vi "Disabled.vi"(7 "Robot Mode":T2, 10 "Match Info":T1={"Autonomous Elapsed Seconds"=0.0, "TeleOp Elapsed Seconds"=0.0, "Disabled Elapsed Seconds"=0.0, "Visited Autonomous"=FALSE, "Visited TeleOp"=FALSE, "Visited Disabled"=FALSE, "Autonomous Settings"={"Autonomous Style"=enum."Independent", "VI Refnum"=refnum}}, 11 "Call Context":T3) -> ()   [LabVIEW 2015]
doc: "This VI is called each time a disabled packet is received from the DS. It is often used to prepare for the next robot mode, to calibrate sensors, etc."
uses:
  <vilib>/Rock Robotics/WPI/DriverStation/WPI_DriverStationDerivedRobotMode.ctl
  <vilib>/Rock Robotics/WPI/DriverStation/WPI_DriverStationRobotMode2.ctl
  <vilib>/Rock Robotics/WPI/DriverStation/WPI_DriverStationMatch Info.ctl
  Drivetrain Code/Drivetrain Control.ctl
  Drivetrain Code/Drivetrain Mode.ctl
  Rollers/Roller Modes.ctl
  Common Code/Auto Roller Commands.ctl
  Common Code/Roller Mode Enum.ctl
  Elevator/Elevator Command.ctl
  Common Code/Change Detect Boolean.vi
  <vilib>/Rock Robotics/WPI/Utilities/WPI_GetSetVariantRefNum.vi
  Robot Global Data.vi
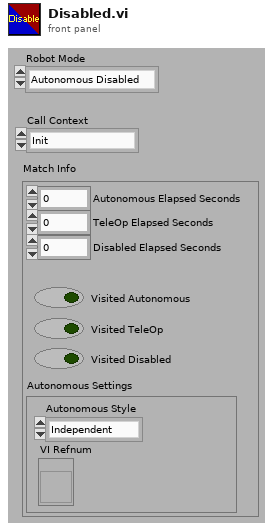
[diagram p1: front panel]
types:
  T1 = typedef "WPI_DriverStationMatch Info.ctl" = cluster{"Autonomous Elapsed Seconds":dbl, "TeleOp Elapsed Seconds":dbl, "Disabled Elapsed Seconds":dbl, "Visited Autonomous":bool, "Visited TeleOp":bool, "Visited Disabled":bool, "Autonomous Settings":cluster{"Autonomous Style":enum16{"Iterative", "Independent"}, "VI Refnum":refnum<vi>}}
  T2 = typedef "WPI_DriverStationRobotMode2.ctl" = enum16{"Autonomous Disabled", "Autonomous Enabled", "Teleop Disabled", "Teleop Enabled", "Disconnected", "Finish", "Test Disabled", "Test Enabled", "Emergency Stopped"}
  T3 = typedef "WPI_DriverStationDerivedRobotMode.ctl" = enum16{"Init", "Execute", "Stop"}
  T4 = enum16{"0", "1", "2", "3", "4", "5", "6", "7", "8", "9", "A", "B", "C", "D", "E", "F", "G", "H", "I", "J", "K", "L", "M", "N", "O", "P", "Q", "R", "S", "T", "U", "V", "W", "X", "Y", "Z", "F1", "F2", "F3", "F4", "F5", "F6", "F7", "F8", "F9", "F10", "F11", "F12", "F13", "F14", "F15", "ADD", "BACK", "BACKSLASH", "CAPITAL", "COMMA", "DECIMAL", "DELETE", "DIVIDE", "DOWN", "END", "EQUALS", "ESCAPE", "GRAVE (`)", "HOME", "INSERT", "LBRACKET", "LCONTROL", "LEFT", "L ALT", "LSHIFT", "LWIN", "MINUS", "MULTIPLY", "NEXT", "NUMLOCK", "NUMPAD_0", "NUMPAD_1", "NUMPAD_2", "NUMPAD_3", "NUMPAD_4", "NUMPAD_5", "NUMPAD_6", "NUMPAD_7", "NUMPAD_8", "NUMPAD_9", "PAUSE", "PERIOD", "PRIOR (PG UP)", "RBRACKET", "RCONTROL", "RETURN", "RIGHT", "R ALT", "RSHIFT", "RWIN", "SCROLL", "SEMICOLON", "SLASH", "SPACE", "SUBTRACT", "TAB", "UP", "ENTER (num pad)", "' (quote)"}
  T5 = typedef "Elevator Command.ctl" = enum16{"Idle", "Load 1", "Load 2", "Load 3", "Drop Stack", "Eject Stack", "Untip Trashcan", "Load Trashcan", "HP Load", "HP Score"}
  T6 = typedef "Auto Roller Commands.ctl" = enum16{"Drag Tote", "Grab Tote", "Idle", "Eject Tote", "Untip Can", "Grab Can"}
  T7 = typedef "Roller Modes.ctl" = cluster{"Auto Roller Command":T6, "Roller Mode":T8, "Override Intake Speed":dbl}
  T8 = typedef "Roller Mode Enum.ctl" = enum16{"Manual", "Safe", "Auto"}
  T9 = typedef "Drivetrain Control.ctl" = cluster{"Mode":T10, "Steer":dbl, "Y":dbl, "Heading Target":dbl, "Strafe X":dbl, "Y Target":dbl, "Strafe Target":dbl, "X Max Speed":dbl, "X Min Speed":dbl, "Y Max Speed":dbl, "Y Min Speed":dbl, "Force strafe":bool, "Pivot Speed":dbl}
  T10 = typedef "Drivetrain Mode.ctl" = enum16{"Manual", "Gyro Steer", "Vision Steer", "Drive Distance", "Yaw Rate Compensate"}
  T11 = typedef "WPI_JoystickDevRef.ctl" = cluster{"Device":T12}
  T12 = typedef "WPI_JoystickDeviceEnum.ctl" = enum16{"USB 0", "USB 1", "USB 2", "USB 3", "USB 4", "USB 5"}
  T13 = typedef "D-Pad.ctl" = cluster{"Top":bool, "Bottom":bool, "None":bool, "Right":bool, "Left":bool}
  T14 = typedef "Button Cluster.ctl" = cluster{"Buttons[0]":bool, "Buttons[1]":bool, "Buttons[2]":bool, "Buttons[3]":bool, "Buttons[4]":bool, "Buttons[5]":bool, "Buttons[6]":bool, "Buttons[7]":bool, "Buttons[8]":bool, "Buttons[9]":bool}
  T15 = typedef "Elevator Mode.ctl" = enum16{"Manual", "Safe", "Auto"}
  T16 = typedef "Elevator Control Command.ctl" = cluster{"Command":T5, "Manual Motor Out":dbl, "Manual Eject Piston":bool, "Mode":T15, "Override Limits":bool, "Manual Stabilizer":bool, "Manual Finger":bool, "Store Trashcan?":bool, "Hold Low?":bool, "Idle Mode":T17, "HP Load":bool, "Unstick":bool, "Raw Height Set":dbl, "Force Store":bool}
  T17 = typedef "Elevator Idle Mode.ctl" = enum16{"Load 1", "Load 2", "Load 3", "Load Can", "Untip Can", "Step Load", "Drop Stack", "Raw Height"}
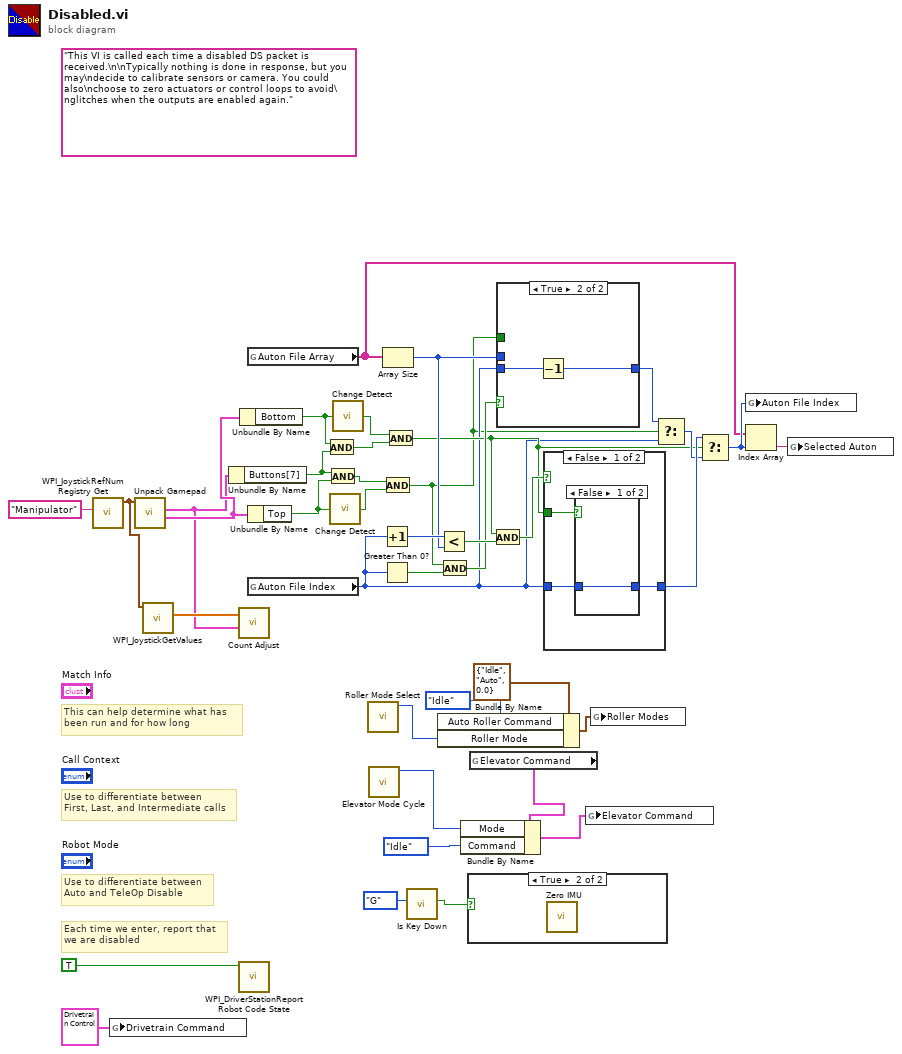
[diagram p0: block diagram]
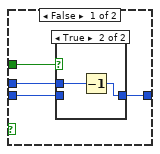
[diagram p3: hidden frame]
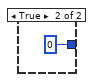
[diagram p5: hidden frame]
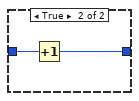
[diagram p6: hidden frame]
diagram:
  (unwired) "This VI is called each time a disabled DS packet is received.\n\nTypically nothing is done in response, but you may\ndecide to calibrate sensors or camera. You could also\nchoose to zero actuators or control loops to avoid\nglitches when the outputs are enabled again."
  # "Each time we enter, report that\nwe are disabled"
  # "Use to differentiate between\nFirst, Last, and Intermediate calls"
  # "This can help determine what has\nbeen run and for how long"
  # "Use to differentiate between\nAuto and TeleOp Disable"
  n1 = call <vilib>:"WPI_JoystickRefNum Registry Get.vi"("refnum name"="Manipulator") -> ("JoystickDevRef"=w6:T11)  [unwired: 9 in, 1 out]
  n2 = global write "Robot Global Data.vi" "Drivetrain Command"(T9 {"Mode"=enum."Manual", "Steer"=0.0, "Y"=0.0, "Heading Target"=0.0, "Strafe X"=0.0, "Y Target"=0.0, "Strafe Target"=0.0, "X Max Speed"=0.0, "X Min Speed"=0.0, "Y Max Speed"=0.0, "Y Min Speed"=0.0, "Force strafe"=FALSE, "Pivot Speed"=0.0} ("Drivetrain Command")) -> ()
  n3 = call "Unpack Gamepad.vi"("JoystickDevRef"=w6) -> ("D-Pad"=w16:T13, "Button Cluster"=w2:T14)  [unwired: 8 in, 1 out]
  n4 = call <vilib>:"WPI_JoystickGetValues.vi"("JoystickDevRef"=w6) -> ("Axes"=w5:dbl[])  [unwired: 6 in, 4 out]
  n5 = Unbundle By Name(w2) -> ("Buttons[7]"=w18:bool)
  n6 = call "Count Adjust.vi"("Button Cluster"=w2, "Axes"=w5) -> ()  [unwired: 10 in]
  n7 = call <vilib>:"WPI_DriverStationReport Robot Code State.vi"("Disabled"=TRUE ("Autonomous")) -> ()  [unwired: 10 in, 1 out]
  n8 = Unbundle By Name(w16) -> ("Bottom"=w15:bool)
  n9 = global read "Robot Global Data.vi" "Auton File Array"() -> (w20:string[])
  n10 = Unbundle By Name(w16) -> ("Top"=w17:bool)
  n11 = global read "Robot Global Data.vi" "Auton File Index"() -> (w22:i32)
  n12 = And(x=w15, y=w18) -> (x .and. y?=w36:bool)
  n13 = And(x=w18, y=w17) -> (x .and. y?=w37:bool)
  n14 = call-poly "Change Detect.vi"("In"=w17) -> ("Changed?"=w23:bool)
  n15 = call-poly "Change Detect.vi"("In"=w15) -> ("Changed?"=w24:bool)
  n16 = call "Roller Mode Select.vi"() -> ("Mode"=w11:T8)  [unwired: 11 in]
  n17 = call "Elevator Mode Cycle.vi"() -> ("Mode"=w9:T15)  [unwired: 11 in]
  n18 = Increment(x=w22) -> (x+1=w35:i32)
  n19 = Greater Than 0?(x=w22) -> (x > 0?=w25:bool)
  n20 = Array Size(array=w20) -> (size(s)=w34:i32)
  n21 = And(x=w37, y=w23) -> (x .and. y?=w14:bool)
  n22 = And(x=w24, y=w36) -> (x .and. y?=w27:bool)
  n23 = call "Is Key Down.vi"("Key"=T4."G") -> ("Key Down?"=w4:bool)  [unwired: 10 in]
  n24 = Bundle By Name(cluster=T7 {"Auto Roller Command"=enum."Idle", "Roller Mode"=enum."Auto", "Override Intake Speed"=0.0} ("Roller Modes"), "Auto Roller Command"=Auto_Roller_Commands."Idle", "Roller Mode"=w11) -> (w10:T7)
  n25 = Less?(x=w35, y=w34) -> (x < y?=w33:bool)
  n26 = And(x=w14, y=w25) -> (x .and. y?=w29:bool)
  n27 = case shown="True" w4 {
    frame False {
    }
    frame True {
      n28 = call "Zero IMU.vi"() -> ()  [unwired: 12 in]
    }
  }
  n29 = global read "Robot Global Data.vi" "Elevator Command"() -> (w1:T16)
  n30 = Bundle By Name(cluster=w1, "Mode"=w9, "Command"=Elevator_Command."Idle") -> (w8:T16)
  n31 = And(x=w27, y=w33) -> (x .and. y?=w32:bool)
  n32 = case shown="True" w29 {
    tunnel: w22 -> [w43 w48]
    tunnel: w14 -> [w42 _]
    tunnel: w34 -> [w41 _]
    tunnel: [w40 w47] -> w28
    frame False {
      n33 = case shown="True" w42 {
        tunnel: [w44 w46] -> w40
        tunnel: w43 -> [w44 _]
        tunnel: w41 -> [_ w45]
        frame False {
        }
        frame True {
          n34 = Decrement(x=w45) -> (x-1=w46:i32)
        }
      }
    }
    frame True {
      n35 = Decrement(x=w48) -> (x-1=w47:i32)
    }
  }
  n36 = case shown="False" w32 {
    tunnel: w22 -> [w51 w55]
    tunnel: w27 -> [w50 _]
    tunnel: [w49 w54] -> w31
    frame False {
      n37 = case shown="False" w50 {
        tunnel: [w52 0 ("Auton File Index")] -> w49
        tunnel: w51 -> [w52 _]
        frame False {
        }
        frame True {
        }
      }
    }
    frame True {
      n38 = Increment(x=w55) -> (x+1=w54:i32)
    }
  }
  n39 = global write "Robot Global Data.vi" "Elevator Command"(w8) -> ()
  n40 = global write "Robot Global Data.vi" "Roller Modes"(w10) -> ()
  n41 = Select(t=w28, s=w14, f=w22) -> (s? t:f=w30:i32)
  n42 = Select(t=w31, s=w27, f=w30) -> (s? t:f=w26:i32)
  n43 = global write "Robot Global Data.vi" "Auton File Index"(w26) -> ()
  n44 = Index Array(array=w20, index=w26) -> (element=w21:string)
  n45 = global write "Robot Global Data.vi" "Selected Auton"(w21) -> ()
